vi "getDeviceType.vi"(8 "error in (no error)":errorcluster, 11 "rfDevice.lvclass in":refnum<class "rfDevice.lvclass">) -> (0 "error out":errorcluster, 2 "type":T1(ring), 3 "rfDevice.lvclass out":refnum<class "rfDevice.lvclass">)   [LabVIEW 2009, in "Tools.lvlib" / "DatabaseHelpers.lvlib" / "rfDevice.lvclass"]
uses:
  rfDevice.lvclass
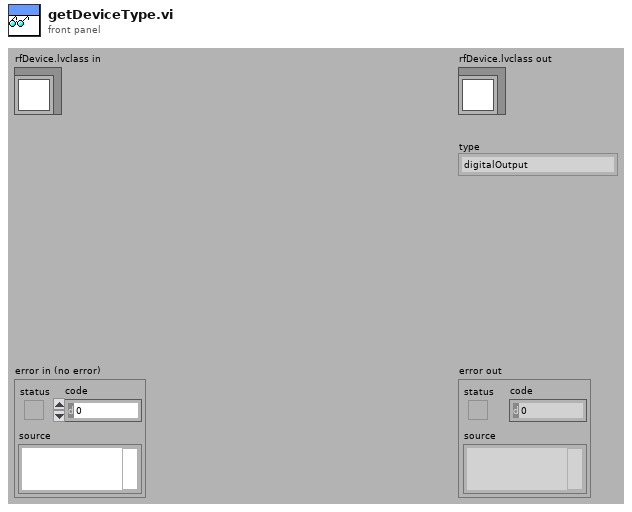
[diagram p1: front panel]
types:
  T1 = enum16{"digitalOutput", "digitalInput", "analogOutput", "analogInput", "rfOutput", "ethernetSupply"}
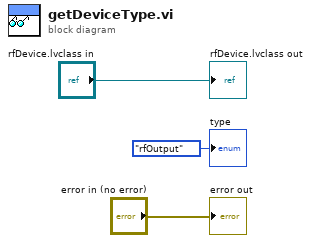
[diagram p0: block diagram]
diagram:
  "error out" <- "error in (no error)"
  "rfDevice.lvclass out" <- "rfDevice.lvclass in"
  "type" <- T1."rfOutput" ("type")
